vi "spiral scan.vi"(10 "maximum frequency":dbl, 11 "scan specification":T1) -> (2 "scan locations":u32[](array[numeric]), 3 "scan specification out":T1)   [LabVIEW 2010]
uses:
  scan_specification_tagResonant.ctl
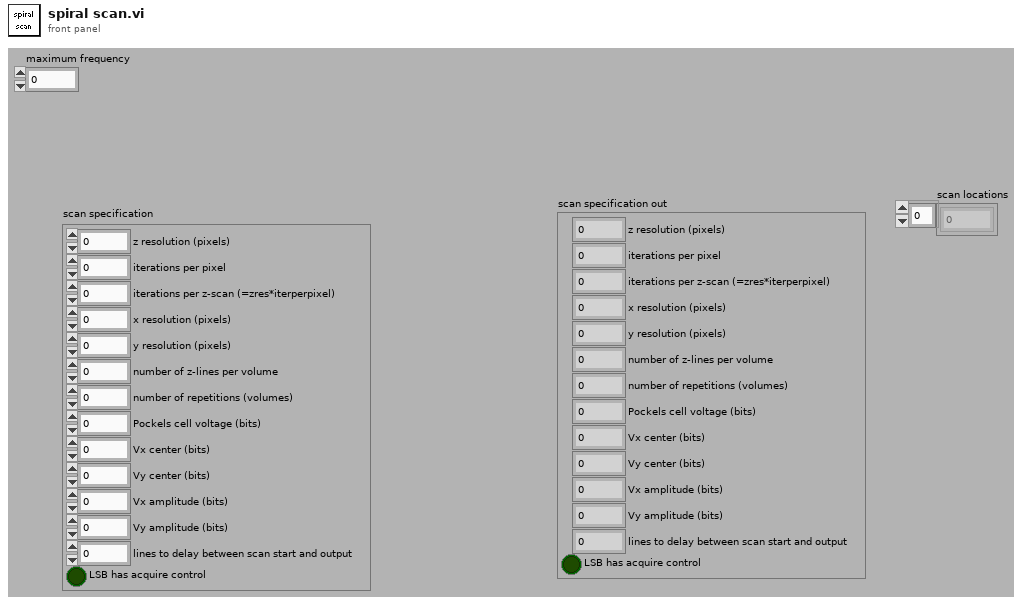
[diagram p1: front panel]
types:
  T1 = typedef "scan_specification_tagResonant.ctl" = cluster{"z resolution (pixels)":u16, "iterations per pixel":u16, "iterations per z-scan (=zres*iterperpixel)":u16, "x resolution (pixels)":u16, "y resolution (pixels)":u16, "number of z-lines per volume":u16, "number of repetitions (volumes)":i32, "Pockels cell voltage (bits)":i16, "Vx center (bits)":i16, "Vy center (bits)":i16, "Vx amplitude (bits)":i16, "Vy amplitude (bits)":i16, "lines to delay between scan start and output":u16, "LSB has acquire control":bool}
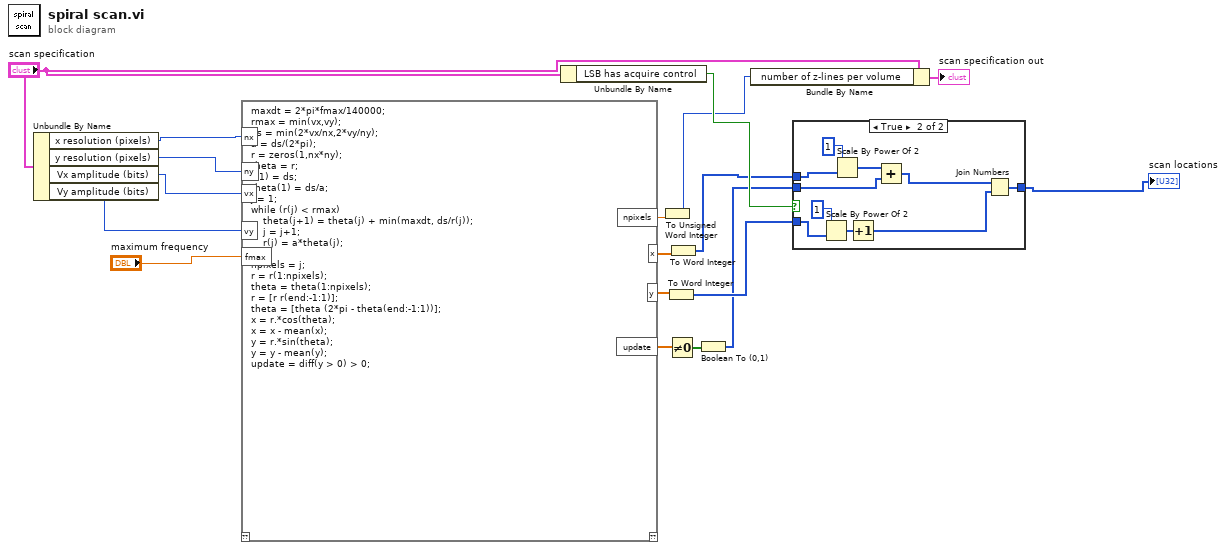
[diagram p0: block diagram]
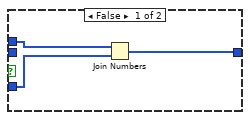
[diagram p2: hidden frame]
diagram:
  n1 = Unbundle By Name("scan specification") -> ("x resolution (pixels)"=w14:u16, "y resolution (pixels)"=w13:u16, "Vx amplitude (bits)"=w12:i16, "Vy amplitude (bits)"=w11:i16)
  n2 = script code="maxdt = 2*pi*fmax/140000;\nrmax = min(vx,vy);\nds = min(2*vx/nx,2*vy/ny);\na = ds/(2*pi);\nr = zeros(1,nx*ny);\ntheta = r;\nr(1) = ds;\ntheta(1) = ds/a;\nj = 1;\nwhile (r(j) < rmax)\n    theta(j+1) = theta(j) + min(maxdt, ds/r(j));\n    j = j+1;\n    r(j) = a*theta(j);\nend\nnpixels = j;\nr = r(1:npixels);\ntheta = theta(1:npixels);\nr = [r r(end:-1:1)];\ntheta = [theta (2*pi - theta(end:-1:1))];\nx = r.*cos(theta);\nx = x - mean(x);\ny = r.*sin(theta);\ny = y - mean(y);\nupdate = diff(y > 0) > 0;"("nx"=w14, "ny"=w13, "vx"=w12, "vy"=w11, "fmax"="maximum frequency") -> ("npixels"=w9:dbl, "x"=w7:dbl[], "y"=w6:dbl[], "update"=w5:dbl[])  [unwired: 1 in, 1 out]
  n3 = Unbundle By Name("scan specification") -> ("LSB has acquire control"=w17:bool)
  n4 = To Unsigned Word Integer(number=w9) -> (unsigned 16bit integer=w8:u16)
  n5 = To Word Integer(number=w6) -> (16bit integer=w2:i16[])
  n6 = Not Equal To 0?(x=w5) -> (x != 0?=w4:bool[])
  n7 = To Word Integer(number=w7) -> (16bit integer=w3:i16[])
  n8 = Boolean To (0,1)(Boolean=w4) -> (0, 1=w1:i16[])
  n9 = Bundle By Name(cluster="scan specification", "number of z-lines per volume"=w8) -> (→"scan specification out":T1)
  n10 = case shown="True" w17 {
    tunnel: w3 -> [w21 w27]
    tunnel: w2 -> [w20 w31]
    tunnel: [w19 w25] -> w15
    tunnel: w1 -> [_ w23]
    frame False {
      n11 = Join Numbers(hi=w21, lo=w20) -> ((hi.lo)=w19:u32[])
    }
    frame True {
      n12 = Scale By Power Of 2(n=1, x=w31) -> (x*2^n=w29:i16[])
      n13 = Scale By Power Of 2(n=1, x=w27) -> (x*2^n=w24:i16[])
      n14 = Increment(x=w29) -> (x+1=w26:i16[])
      n15 = Add(x=w24, y=w23) -> (x+y=w22:i16[])
      n16 = Join Numbers(hi=w22, lo=w26) -> ((hi.lo)=w25:u32[])
    }
  }
  "scan locations" <- w15
